vi "内泄露.vi"(0 "曲线引用":refnum<vi>, 1 "内泄露":cluster{"下限":dbl, "上限":dbl}, 3 "错误输入":errorcluster) -> (7 "曲线引用输出":refnum<vi>, 8 "OK？":bool, 10 "错误输出":errorcluster)   [LabVIEW 2017]
uses:
  <userlib>/_MGI/1D Array/MGI Average/MGI Average (DBL[]).vi
  Global_Variable/Global.vi
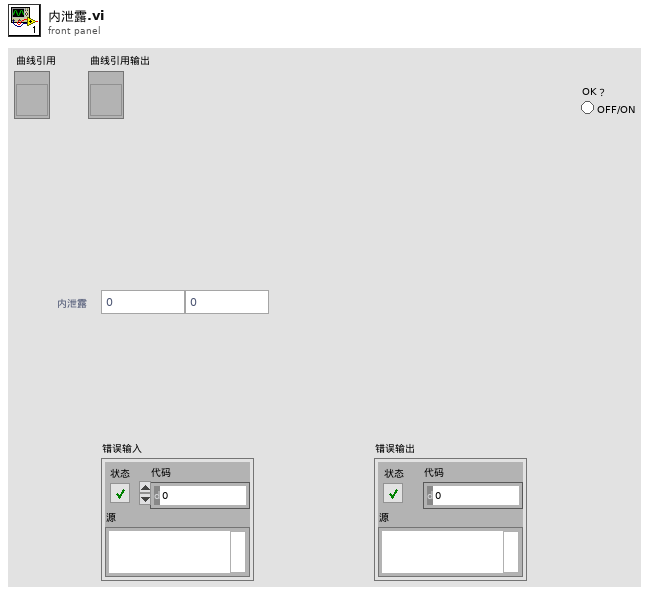
[diagram p1: front panel]
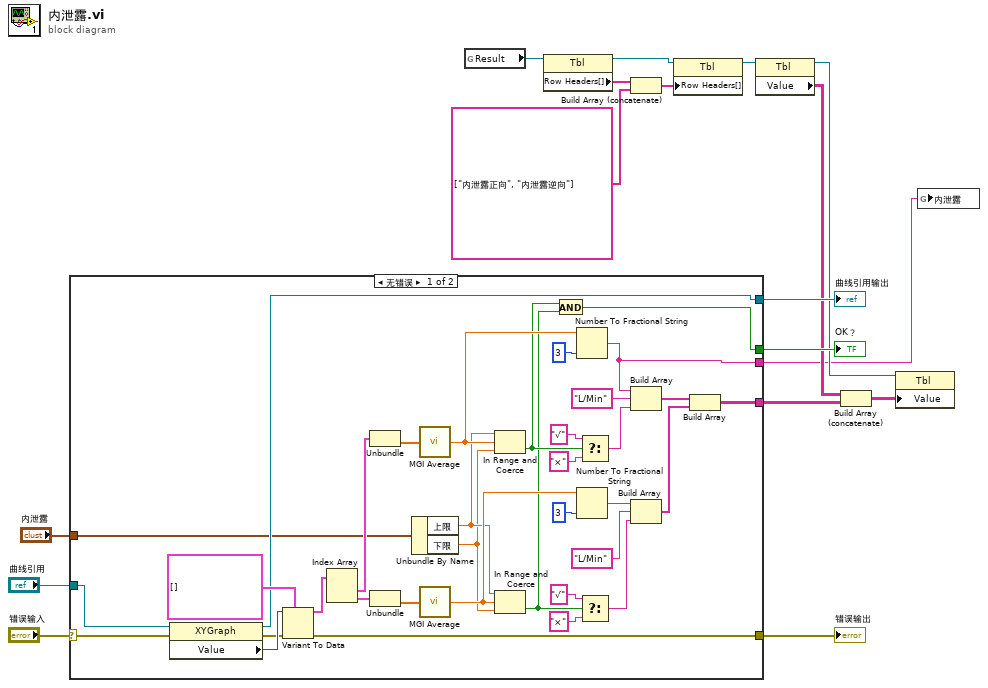
[diagram p0: block diagram]
diagram:
  n1 = case shown="无错误" "错误输入" {
    selector: "错误输入" -> [w50 w54]
    tunnel: [w47 w54] -> w16
    tunnel: "曲线引用" -> [w46 w53]
    tunnel: [w49 w53] -> w14
    tunnel: [w19 _] -> w13
    tunnel: "内泄露" -> [w35 _]
    tunnel: [w36 _] -> w9
    tunnel: [w18 _] -> w1
    frame No Error {
      n2 = property class="XYGraph"(reference=w46, error in=w50) -> (reference out=w49:refnum<vi>, error out=w48:errorcluster, "Value"=w52:variant)
      n3 = Variant To Data(error in=w48, type=cluster{dbl[], dbl[]}[] [], Variant=w52) -> (data=w40:cluster{dbl[], dbl[]}[], error out=w47:errorcluster)
      n4 = Index Array(array=w40) -> (element #1=w39:cluster{dbl[], dbl[]}, element #2=w38:cluster{dbl[], dbl[]})  [unwired: 2 in]
      n5 = Unbundle(w39) -> (w33:dbl[])  [unwired: 1 out]
      n6 = Unbundle(w38) -> (w25:dbl[])  [unwired: 1 out]
      n7 = Unbundle By Name(w35) -> ("上限"=w24:dbl, "下限"=w23:dbl)
      n8 = call-poly <userlib>:"MGI Average.vi"("Double[]"=w33) -> ("Average"=w34:dbl)  [unwired: 1 in]
      n9 = call-poly <userlib>:"MGI Average.vi"("Double[]"=w25) -> ("Average"=w32:dbl)  [unwired: 1 in]
      n10 = In Range and Coerce(upper limit=w24, x=w34, lower limit=w23) -> (In Range?=w21:bool)  [unwired: 1 out]
      n11 = In Range and Coerce(upper limit=w24, x=w32, lower limit=w23) -> (In Range?=w20:bool)  [unwired: 1 out]
      n12 = And(x=w21, y=w20) -> (x .and. y?=w19:bool)
      n13 = Number To Fractional String(number=w34, precision (6)=i16 3 ("精度(6)")) -> (F-format string=w18:string)  [unwired: 2 in]
      n14 = Number To Fractional String(number=w32, precision (6)=i16 3 ("精度(6)")) -> (F-format string=w27:string)  [unwired: 2 in]
      n15 = Select(t="√" ("元素"), s=w21, f="×" ("元素")) -> (s? t:f=w41:string)
      n16 = Select(t="√" ("元素"), s=w20, f="×" ("元素")) -> (s? t:f=w31:string)
      n17 = Build Array(w18, "L/Min" ("元素"), w41) -> (w37:string[])
      n18 = Build Array(w27, "L/Min" ("元素"), w31) -> (w22:string[])
      n19 = Build Array(w37, w22) -> (w36:string[][])
    }
    frame Error {
    }
  }
  "错误输出" <- w16
  "曲线引用输出" <- w14
  "OK？" <- w13
  n20 = global read "Global.vi" "Result"() -> (w8:refnum<vi>)
  n21 = property class="Tbl"(reference=w8) -> (reference out=w7:refnum<vi>, "Row Headers[]"=w5:string[])  [unwired: 1 in, 1 out]
  n22 = Build Array (concatenate)(w5, string[] ["内泄露正向", "内泄露逆向"] ("列首字符串[]")) -> (w3:string[])
  n23 = property class="Tbl"(reference=w7, "Row Headers[]"=w3) -> (reference out=w6:refnum<vi>)  [unwired: 1 in, 1 out]
  n24 = property class="Tbl"(reference=w6) -> (reference out=w12:refnum<vi>, "Value"=w11:string[][])  [unwired: 1 in, 1 out]
  n25 = Build Array (concatenate)(w11, w9) -> (w10:string[][])
  n26 = property class="Tbl"(reference=w12, "Value"=w10) -> ()  [unwired: 1 in, 2 out]
  n27 = global write "检测结果.vi" "内泄露"(w1) -> ()
